vi "Set_subDir_Data.vi"(8 "error in (no error)":errorcluster, 10 "data":T1, 11 "AB_Dest_SubDir in":refnum<class "AB_Dest_SubDir.lvclass">) -> (0 "error out":errorcluster, 3 "AB_Dest_SubDir out":refnum<class "AB_Dest_SubDir.lvclass">)   [LabVIEW 2020, in "AB_Dest_SubDir.lvclass"]
uses:
  <vilib>/AppBuilder/AB_Classes/Destination/Dest_SubDirectory/AB_Dest_SubDir.lvclass
  <vilib>/AppBuilder/AB_Classes/Destination/Dest_SubDirectory/AB_SubDirectory.ctl
  <vilib>/AppBuilder/AB_Classes/Destination/Dest_SubDirectory/AB_Dest_SubDir.lvclass/AB_Dest_SubDir.ctl
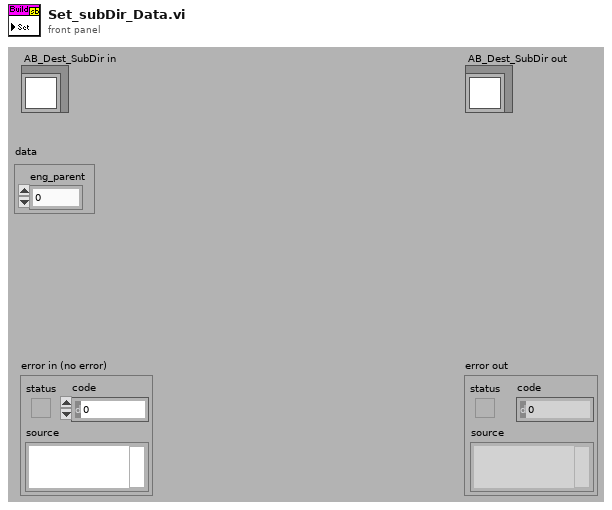
[diagram p1: front panel]
types:
  T1 = typedef "AB_SubDirectory.ctl" = cluster{"eng_parent":i32}
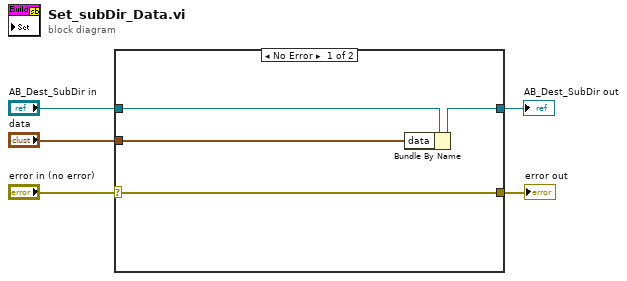
[diagram p0: block diagram]
diagram:
  n1 = case shown="No Error" "error in (no error)" {
    selector: "error in (no error)" -> [w9 w11]
    tunnel: [w9 w11] -> w4
    tunnel: "AB_Dest_SubDir in" -> [w8 w10]
    tunnel: [w7 w10] -> w2
    tunnel: "data" -> [w6 _]
    frame No Error {
      n2 = Bundle By Name(cluster=w8, "data"=w6) -> (w7:refnum<class "AB_Dest_SubDir.lvclass">)
    }
    frame Error {
    }
  }
  "error out" <- w4
  "AB_Dest_SubDir out" <- w2
